vi "TranslatorBooster DataType Decode.vi"(11 "DataType Encoded":string) -> (3 "DataType Decoded":string)   [LabVIEW 2014, in "Complex Numbers.lvlib"]
uses:
  <vilib>/Aledyne-TSXperts/Arduino Compatible Compiler for LabVIEW/addons/Complex Numbers/Complex Numbers.lvlib
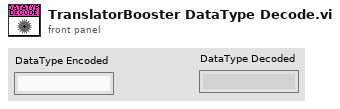
[diagram p1: front panel]
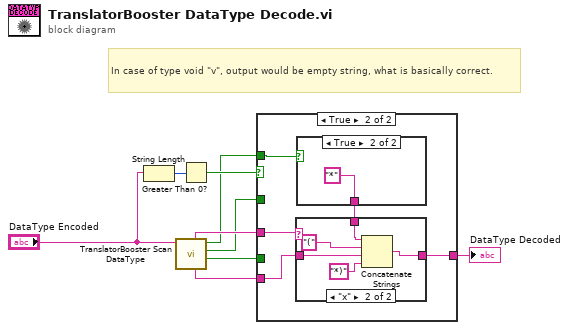
[diagram p0: block diagram]
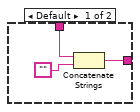
[diagram p3: hidden frame]
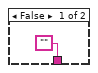
[diagram p4: hidden frame]
diagram:
  # "In case of type void \"v\", output would be empty string, what is basically correct."
  n1 = String Length(string="DataType Encoded") -> (length=w7:i32)
  n2 = call <vilib>:"TranslatorBooster Scan DataType.vi"("whole match"="DataType Encoded") -> ("usnigned?"=w4:bool, "ref?"=w3:bool, "pointer?"=w2:bool, "dataType"=w5:string, "type"=w6:string)  [unwired: 6 in]
  n3 = Greater Than 0?(x=w7) -> (x > 0?=w9:bool)
  n4 = case shown="True" w9 {
    tunnel: w2 -> [_ w14]
    tunnel: w3 -> [_ _]
    tunnel: w4 -> [_ _]
    tunnel: w5 -> [_ w13]
    tunnel: w6 -> [_ w11]
    tunnel: [_ w10] -> w1
    frame False {
    }
    frame True {
      n5 = case shown="True" w14 {
        tunnel: ["" "*"] -> w12
        frame False {
        }
        frame True {
        }
      }
      n6 = case shown="\"x\"" w11 {
        tunnel: w13 -> [_ w20]
        tunnel: w12 -> [w17 w19]
        tunnel: [w15 w18] -> w10
        frame Default {
          n7 = Concatenate Strings(w17, "") -> (w15:string)
        }
        frame "x" {
          n8 = Concatenate Strings(w19, "(" ("string"), w20, "*)" ("string")) -> (w18:string)
        }
      }
    }
  }
  "DataType Decoded" <- w1
